vi "Read Waveform Number of Elements.vi"(11 "AO in":refnum<class "Analog Output.lvclass">) -> (3 "number of elements":u16)   [LabVIEW 2017, in "Analog IO.lvlib" / "Analog Output.lvclass"]
uses:
  Analog Output.lvclass
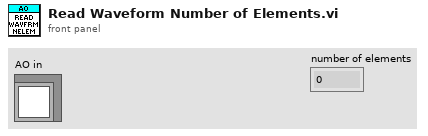
[diagram p1: front panel]
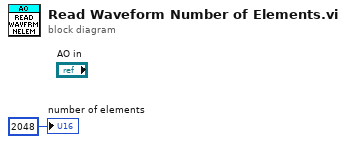
[diagram p0: block diagram]
diagram:
  "number of elements" <- u16 2048 ("number of elements")
